vi "Event Current State.vi"(8 "error in":errorcluster, 10 "Current State":string, 11 "Context in":refnum<class "Context.lvclass">) -> (0 "error out":errorcluster, 3 "Context out":refnum<class "Context.lvclass">)   [LabVIEW 2021, in "Context.lvlib" / "Context.lvclass"]
uses:
  Context.lvclass
  Context.lvclass/Context.ctl
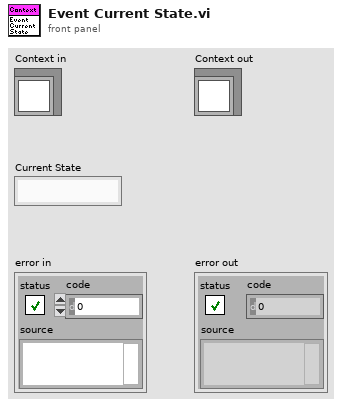
[diagram p1: front panel]
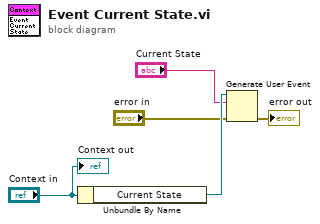
[diagram p0: block diagram]
diagram:
  n1 = Unbundle By Name("Context in") -> ("Current State"=w4:refnum<user-event>)
  n2 = Generate User Event(user event=w4, event data cluster="Current State", error in="error in") -> (error out=→"error out":errorcluster)  [unwired: 1 in, 1 out]
  "Context out" <- "Context in"
